vi "find_circles test.vi"() -> ()   [LabVIEW 2017]
uses:
  <vilib>/vision/NI_Vision_Development_Module.lvlib
  find_circles parameters.ctl
  Vision.lvlib
panel:
  in  "Field of View":cluster{"fieldOfViewX":sgl, "fieldOfViewY":sgl}={"fieldOfViewX"=1.4, "fieldOfViewY"=1.048}
  in  "find_circles parameters":T1={"minRadius"=0.1, "maxRadius"=1.0, "houghGradientParam1"=100, "houghGradientParam2"=50}
  out "Circles":T2(array[cluster])
  out "Number of Circles":i32
  in  "File Path":path=path "C:/Users/cfang/Dropbox/TFPX Heater GM0108 - Gantry Camera/sample_03.png"
  out "error out":errorcluster
  out "Image":T3(plugin-control)
  in  "debug":bool
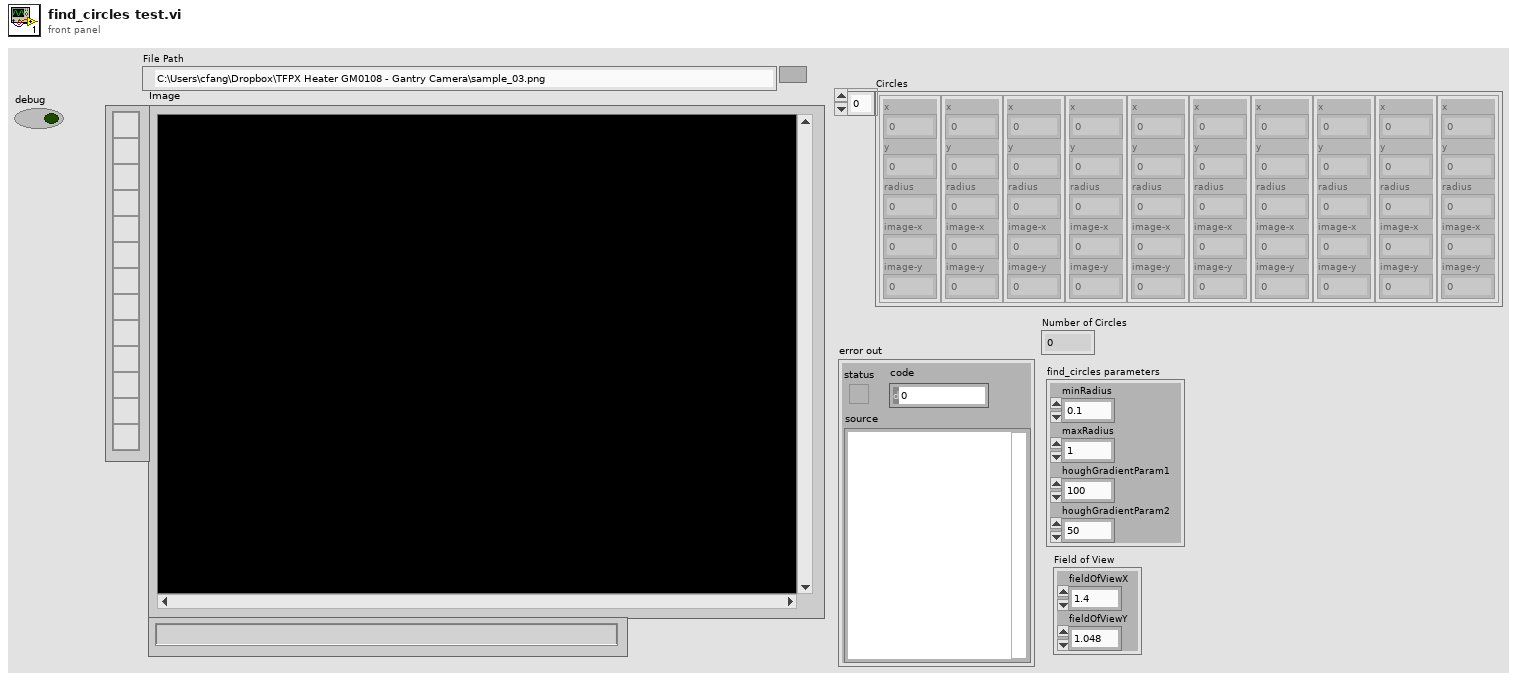
[diagram p1: front panel]
types:
  T1 = typedef "Vision.lvlib/find_circles parameters.ctl" = cluster{"minRadius":sgl, "maxRadius":sgl, "houghGradientParam1":i32, "houghGradientParam2":i32}
  T2 = cluster{"x":dbl, "y":dbl, "radius":dbl, "image-x":dbl, "image-y":dbl}[]
  T3 = typedef "IMAQ Image.ctl" = refnum<image>
  T4 = typedef "Image Type" = u32
  T5 = cluster{"Left":i32, "Top":i32, "Right":i32, "Bottom":i32}
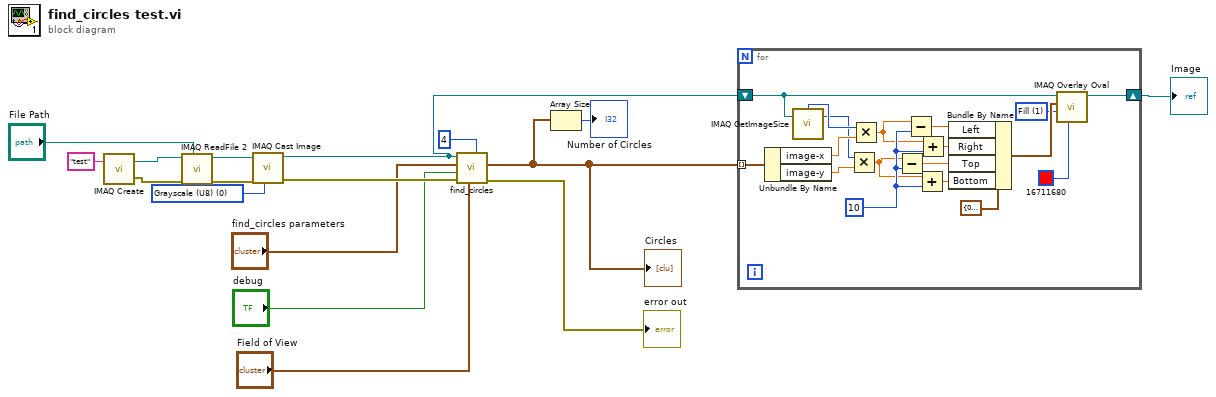
[diagram p0: block diagram]
diagram:
  w11 = T4 0 items=["Grayscale (U8)", "Grayscale (I16)", "Grayscale (SGL)", "Complex (CSG)", "RGB (U32)", "HSL (U32)", "RGB (U64)", "Grayscale (U16)"] ("Image Type")
  n1 = call "IMAQ Create"("Image Name"="test") -> ("New Image"=w17:T3, "error out"=w15:errorcluster)  [unwired: 4 in]
  n2 = call "IMAQ ReadFile 2"("File Path"="File Path", "error in (no error)"=w15, "Image"=w17) -> ("error out"=w13:errorcluster, "Image Out"=w12:T3)  [unwired: 4 in, 3 out]
  n3 = call "IMAQ Cast Image"("Image Type"=w11, "error in (no error)"=w13, "Image Src"=w12) -> ("error out"=w8:errorcluster, "Image Dst Out"=w2:T3)  [unwired: 7 in]
  n4 = call "find_circles.vi"("shrinkFactor"=4 ("Shrink Factor"), "Field of View"="Field of View", "error in"=w8, "debug"="debug", "find_circles parameters"="find_circles parameters", "Image"=w2) -> ("error out"=→"error out":errorcluster, "Circles"=w3:T2)  [unwired: 4 in]
  "Circles" <- w3
  n5 = Array Size(array=w3) -> (size(s)=→"Number of Circles":i32)
  n6 = for {
    tunnel: w3 -> [w35] mode=indexing
    shift-right: [w19] -> w1
    shift-left: w2 -> [w30]
    w18 = u32 1 items=["Frame", "Fill"] ("Drawing Mode (Frame)")
    w23 = 10
    n7 = Unbundle By Name(w35) -> ("image-x"=w34:dbl, "image-y"=w32:dbl)
    n8 = call "IMAQ GetImageSize"("Image"=w30) -> ("Y Resolution"=w31:i32, "X Resolution"=w33:i32)  [unwired: 3 in, 1 out]
    n9 = Multiply(x=w31, y=w32) -> (x*y=w22:dbl)
    n10 = Multiply(x=w33, y=w34) -> (x*y=w21:dbl)
    n11 = Subtract(x=w22, y=w23) -> (x-y=w24:dbl)
    n12 = Subtract(x=w21, y=w23) -> (x-y=w25:dbl)
    n13 = Add(x=w22, y=w23) -> (x+y=w26:dbl)
    n14 = Add(x=w21, y=w23) -> (x+y=w27:dbl)
    n15 = Bundle By Name(cluster=T5 {"Left"=0, "Top"=0, "Right"=0, "Bottom"=0} ("Bounding Rectangle"), "Left"=w25, "Right"=w27, "Top"=w24, "Bottom"=w26) -> (w20:T5)
    n16 = call "IMAQ Overlay Oval"("Color"=u32 16711680, "Drawing Mode (Frame)"=w18, "Bounding Rectangle"=w20, "Image"=w30) -> ("Image Out"=w19:T3)  [unwired: 6 in, 1 out]
  }
  "Image" <- w1
